vi "Move Out Previous Page.vi"(8 "error in (no error)":errorcluster, 11 "Project View in":refnum<class "Project View.lvclass">) -> (0 "error out":errorcluster, 3 "Project View out":refnum<class "Project View.lvclass">)   [LabVIEW 2013, in "Project View.lvlib" / "Project View.lvclass"]
uses:
  Project View.lvclass
  Project View.lvclass/Project View.ctl
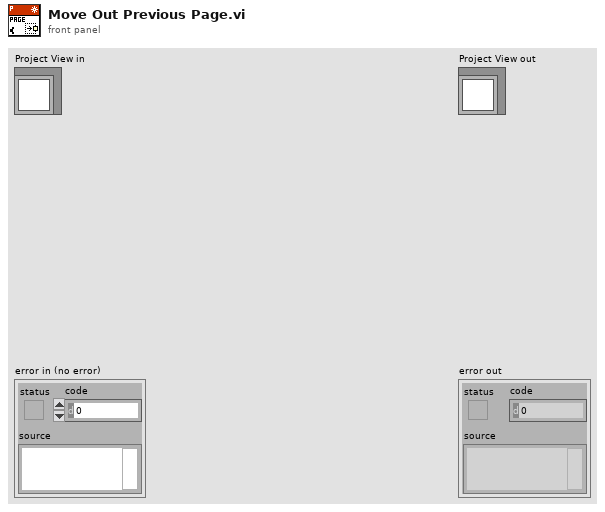
[diagram p1: front panel]
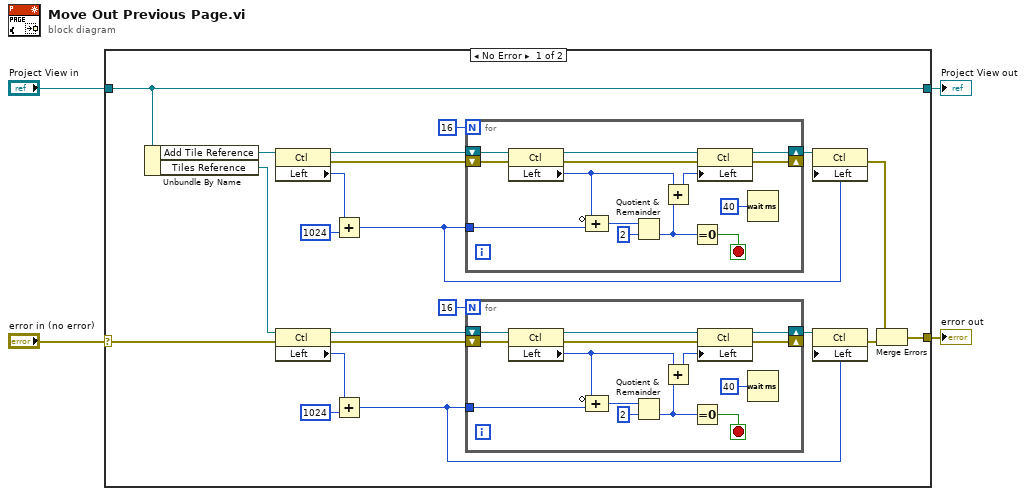
[diagram p0: block diagram]
diagram:
  n1 = case shown="No Error" "error in (no error)" {
    selector: "error in (no error)" -> [w15 w55]
    tunnel: "Project View in" -> [w9 w54]
    tunnel: [w11 w55] -> w2
    tunnel: [w9 w54] -> w3
    frame No Error {
      n2 = Unbundle By Name(w9) -> ("Add Tile Reference"=w23:refnum<vi>, "Tiles Reference"=w16:refnum<vi>)
      n3 = property class="Ctl"(reference=w23) -> (reference out=w25:refnum<vi>, error out=w13:errorcluster, "Left"=w22:i32)  [unwired: 1 in]
      n4 = property class="Ctl"(reference=w16, error in=w15) -> (reference out=w17:refnum<vi>, error out=w14:errorcluster, "Left"=w19:i32)
      n5 = Add(x=w22, y=1024 ("Position:Left")) -> (x+y=w6:i32)
      n6 = Add(x=w19, y=1024 ("Position:Left")) -> (x+y=w5:i32)
      n7 = for {
        N: 16 -> [_]
        shift-right: [w51] -> w21
        shift-left: w25 -> [w53]
        shift-right: [w44] -> _
        shift-left: w13 -> [w52]
        tunnel: w6 -> [w40]
        stop <- w43 stop-if-true
        n8 = property class="Ctl"(reference=w53, error in=w52) -> (reference out=w49:refnum<vi>, error out=w50:errorcluster, "Left"=w41:i32)
        n9 = Compound Arithmetic op=ADD(invert w41, w40) -> (w47:i32)
        n10 = Quotient & Remainder(x=w47, y=2) -> (floor(x/y)=w45:i32)  [unwired: 1 out]
        n11 = Add(x=w41, y=w45) -> (x+y=w48:i32)
        n12 = Equal To 0?(x=w45) -> (x = 0?=w43:bool)
        n13 = property class="Ctl"(reference=w49, error in=w50, "Left"=w48) -> (reference out=w51:refnum<vi>, error out=w44:errorcluster)
        n14 = Wait (ms)(milliseconds to wait=u32 40) -> ()  [unwired: 1 out]
      }
      n15 = for {
        N: 16 -> [_]
        shift-right: [w37] -> w20
        shift-left: w17 -> [w39]
        shift-right: [w30] -> _
        shift-left: w14 -> [w38]
        tunnel: w5 -> [w26]
        stop <- w29 stop-if-true
        n16 = property class="Ctl"(reference=w39, error in=w38) -> (reference out=w35:refnum<vi>, error out=w36:errorcluster, "Left"=w27:i32)
        n17 = Compound Arithmetic op=ADD(invert w27, w26) -> (w33:i32)
        n18 = Quotient & Remainder(x=w33, y=2) -> (floor(x/y)=w31:i32)  [unwired: 1 out]
        n19 = Add(x=w27, y=w31) -> (x+y=w34:i32)
        n20 = Equal To 0?(x=w31) -> (x = 0?=w29:bool)
        n21 = property class="Ctl"(reference=w35, error in=w36, "Left"=w34) -> (reference out=w37:refnum<vi>, error out=w30:errorcluster)
        n22 = Wait (ms)(milliseconds to wait=u32 40) -> ()  [unwired: 1 out]
      }
      n23 = property class="Ctl"(reference=w21, "Left"=w6) -> (error out=w10:errorcluster)  [unwired: 1 in, 1 out]
      n24 = property class="Ctl"(reference=w20, "Left"=w5) -> (error out=w12:errorcluster)  [unwired: 1 in, 1 out]
      n25 = Merge Errors(w10, w12) -> (w11:errorcluster)
    }
    frame Error {
    }
  }
  "error out" <- w2
  "Project View out" <- w3
